vi "Receive Page.vi"(8 "error in (no error)":errorcluster, 11 "Node Ptr":T1 format="%.0x") -> (0 "error out":errorcluster)   [LabVIEW 2018, in "Vires VTD System Explorer.lvlib"]
uses:
  Vires VTD System Explorer.lvlib
  <vilib>/NI Veristand/Custom Device API/Custom Device Item Ref.ctl
  <vilib>/NI Veristand/Custom Device API/Custom Device Channel.ctl
  <vilib>/NI Veristand/Custom Device API/Custom Device Channel Type.ctl
  Shared/Constants.vi
  <vilib>/NI Veristand/Custom Device API/Custom Device API.lvlib
  Shared/Vires VTD Shared.lvlib
panel:
  in  "PlayerID":u8=1
  in  "RDB Receive Objects":string caption="RDB Object Name"
  in  "Add to Outputs":bool
  in  "Tree":string(tree)
  in  "Header":cluster{"Section Name":string}={"Section Name"="Custom Device Item Settings"}
  in  "Description":string
  in  "Name":string
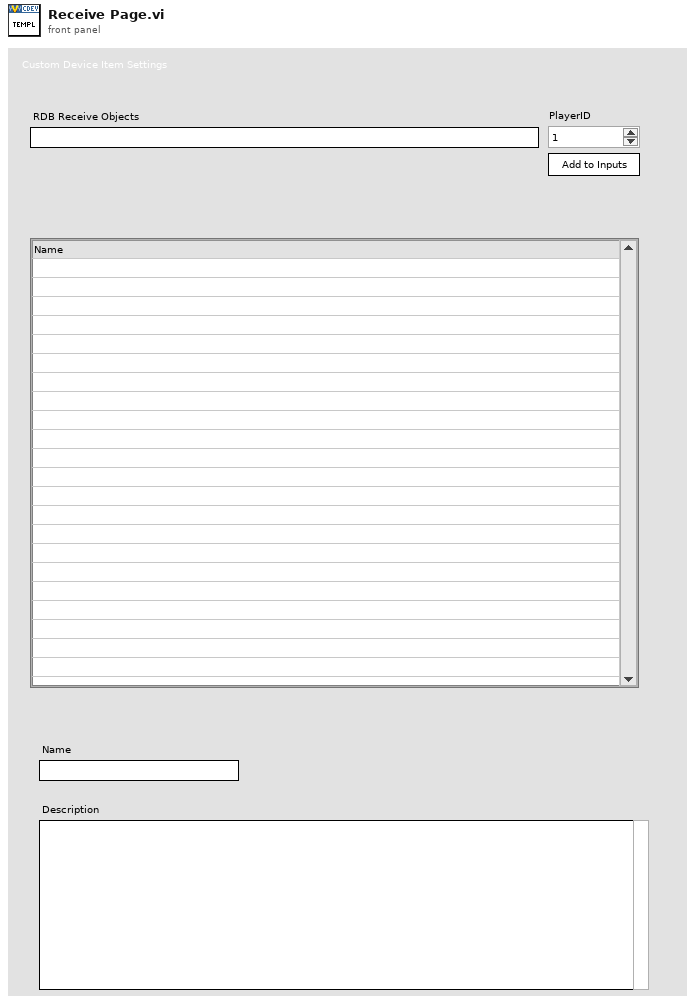
[diagram p1: front panel]
types:
  T1 = typedef "Custom Device API.lvlib/Custom Device Item Ref.ctl" = u64
  T2 = typedef "Custom Device API.lvlib/Custom Device Item Info.ctl" = cluster{"Name":string, "Is Channel":bool, "GUID":string, "Is Waveform":bool}
  T3 = typedef "Custom Device API.lvlib/Custom Device Channel.ctl" = cluster{"Type":T4, "Units":string, "Default Value":dbl, "Faultable":bool, "Scalable":bool}
  T4 = typedef "Custom Device API.lvlib/Custom Device Channel Type.ctl" = enum16{"Input", "Output"}
  T5 = typedef "Custom Device API.lvlib/Custom Device Commands.ctl" = enum16{"Default", "Item renamed", "Shutdown", "Dynamic button pressed"}
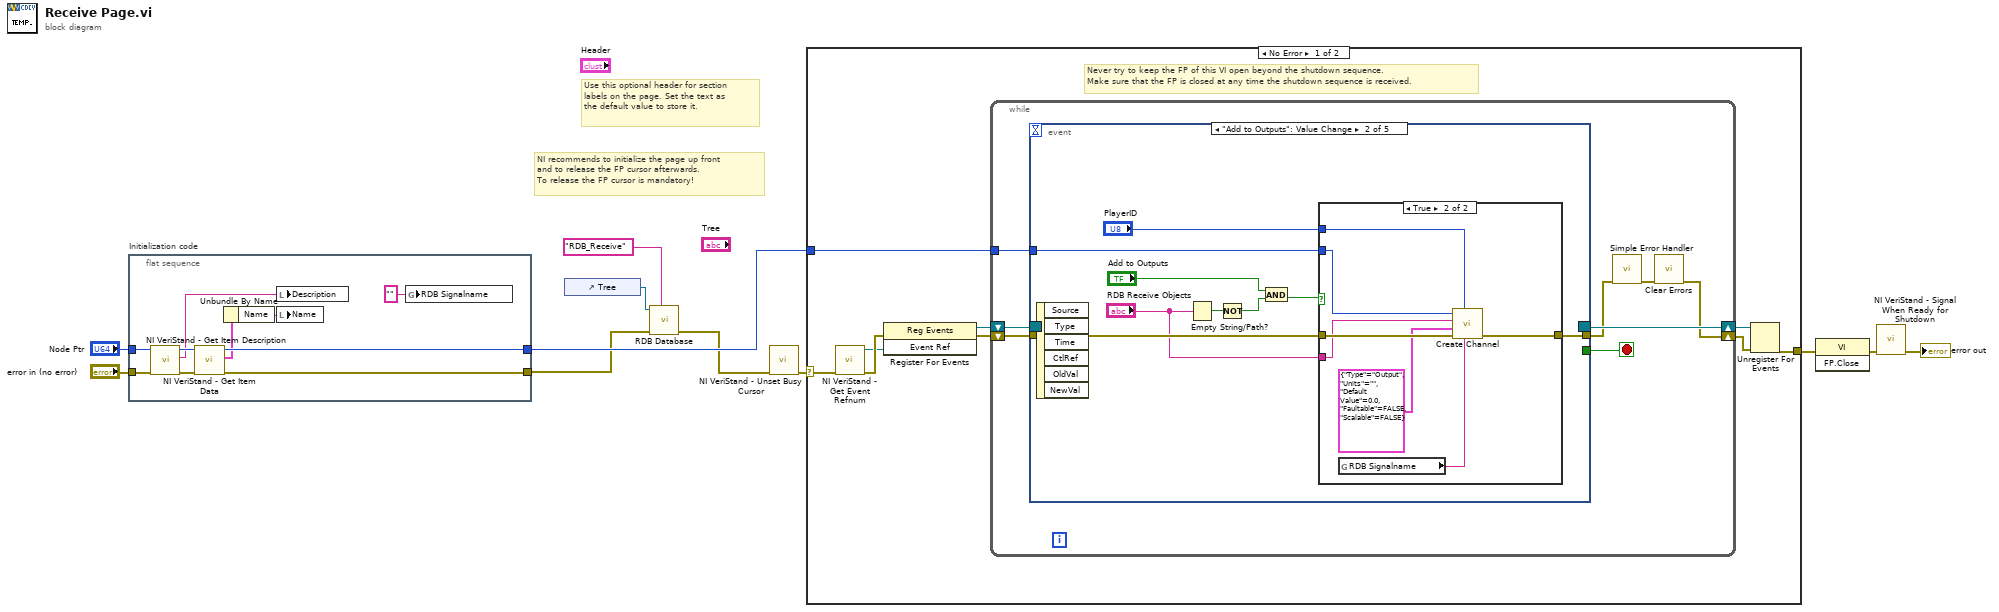
[diagram p0: block diagram]
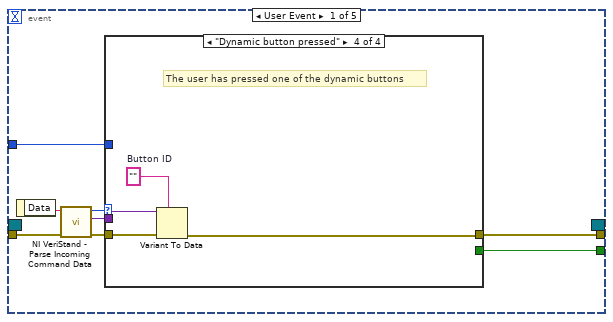
[diagram p2: hidden frame]
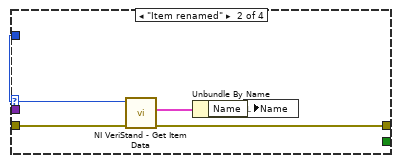
[diagram p4: hidden frame]
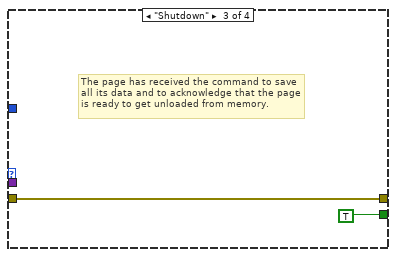
[diagram p5: hidden frame]
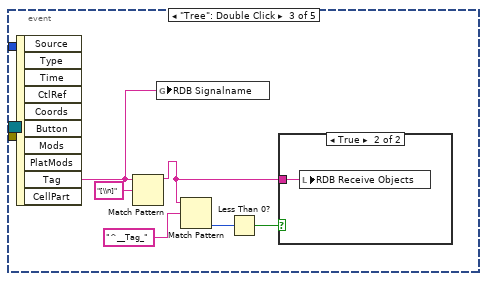
[diagram p7: hidden frame]
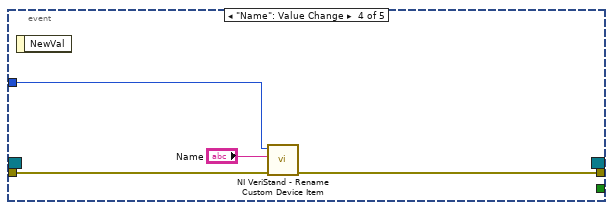
[diagram p9: hidden frame]
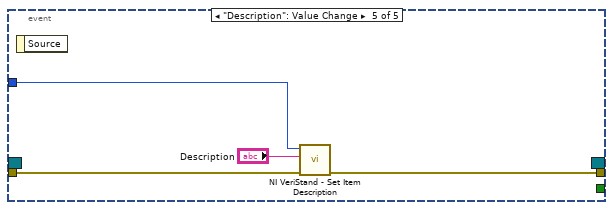
[diagram p10: hidden frame]
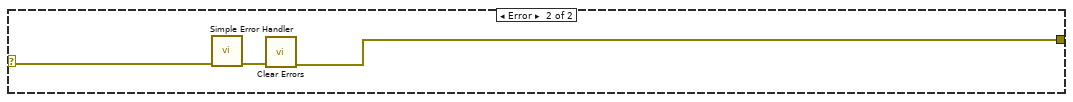
[diagram p11: hidden frame]
diagram:
  # "Use this optional header for section labels on the page. Set the text as the default value to store it."
  # "NI recommends to initialize the page up front\nand to release the FP cursor afterwards.\nTo release the FP cursor is mandatory!"
  n1 = flat-sequence "Initialization code" {
    tunnel: "error in (no error)" -> [w19]
    tunnel: "Node Ptr" -> [w18]
    tunnel: [w13] -> w4
    tunnel: [w21] -> w5
    frame #0 {
      n2 = call <vilib>:"NI VeriStand - Get Item Description.vi"("error in (no error)"=w19, "Item Ref in"=w18) -> ("error out"=w16:errorcluster, "Description"=w17:string, "Item Ref out"=w20:T1)  [unwired: 7 out]
      n3 = call <vilib>:"NI VeriStand - Get Item Data.vi"("error in (no error)"=w16, "Item Ref in"=w20) -> ("error out"=w13:errorcluster, "Item Info"=w15:T2, "Item Ref out"=w21:T1)  [unwired: 7 out]
      n4 = Unbundle By Name(w15) -> ("Name"=w14:string)
      n5 = local write "Description"(w17) -> ()
      n6 = local write "Name"(w14) -> ()
      n7 = global write "Constants.vi" "RDB Signalname"("" ("RDB Signalname")) -> ()
    }
  }
  n8 = control-ref of="Tree"() -> (w3:refnum<vi>)
  n9 = call "RDB Database.vi"("Filter Cluster"="RDB_Receive", "error in (no error)"=w4, "reference"=w3) -> ("error out"=w2:errorcluster)  [unwired: 8 in]
  n10 = call <vilib>:"NI VeriStand - Unset Busy Cursor.vi"("error in (no error)"=w2) -> ("error out"=w7:errorcluster)  [unwired: 10 out]
  n11 = case shown="No Error" w7 {
    selector: w7 -> [w22 w93]
    tunnel: [w27 w91] -> w11
    tunnel: w5 -> [w23 _]
    frame No Error {
      # "Never try to keep the FP of this VI open beyond the shutdown sequence.\nMake sure that the FP is closed at any time the shutdown sequence is received."
      n12 = call <vilib>:"NI VeriStand - Get Event Refnum.vi"("error in (no error)"=w22) -> ("error out"=w30:errorcluster, "Event Ref"=w26:refnum<user-event>)  [unwired: 9 out]
      n13 = register-events(error in=w30, w26) -> (reference out=w24:refnum<event-registration>, error out=w25:errorcluster)  [unwired: 1 in]
      n14 = while {
        tunnel: w23 -> [w34]
        shift-right: [w31] -> w28
        shift-left: w25 -> [w37]
        shift-right: [w38] -> w29
        shift-left: w24 -> [w36]
        stop <- w35 stop-if-true
        n15 = event shown="[1] \"Add to Outputs\": Value Change" {
          selector: w36 -> [_ _ _ _ _]
          dyn-events: [_ _ _ _ _] -> w38
          timeout: _ -> [_ _ _ _ _]
          tunnel: w37 -> [w46 w62 _ w86 w89]
          tunnel: [w42 _ _ _ _] -> w35
          tunnel: [w41 w60 _ w85 w88] -> w33
          tunnel: w34 -> [w40 w63 _ w84 w90]
          event User Event {
            n16 = event-data() -> ("Data"=w45:string)  [unwired: 1 out]
            n17 = call <vilib>:"NI VeriStand - Parse Incoming Command Data.vi"("error in (no error)"=w46, "Incoming data"=w45) -> ("error out"=w44:errorcluster, "Outgoing data"=w39:variant, "Action"=w43:T5)  [unwired: 7 out]
            n18 = case shown="\"Dynamic button pressed\"" w43 {
              tunnel: w44 -> [w47 w52 w53 w58]
              tunnel: [_ _ TRUE _] -> w42
              tunnel: [w47 w49 w53 w55] -> w41
              tunnel: w40 -> [_ w51 _ _]
              tunnel: w39 -> [_ _ _ w57]
              frame "Default", Default {
              }
              frame "Item renamed" {
                n19 = call <vilib>:"NI VeriStand - Get Item Data.vi"("error in (no error)"=w52, "Item Ref in"=w51) -> ("error out"=w49:errorcluster, "Item Info"=w50:T2)  [unwired: 8 out]
                n20 = Unbundle By Name(w50) -> ("Name"=w48:string)
                n21 = local write "Name"(w48) -> ()
              }
              frame "Shutdown" {
                # "The page has received the command to save all its data and to acknowledge that the page is ready to get unloaded from memory."
              }
              frame "Dynamic button pressed" {
                w56 = ""  # Button ID
                # "The user has pressed one of the dynamic buttons"
                n22 = Variant To Data(error in=w58, type=w56, Variant=w57) -> (error out=w55:errorcluster)  [unwired: 1 out]
              }
            }
          }
          event "Add to Outputs": Value Change {
            n23 = event-data() -> ()  [unwired: 7 out]
            n24 = Empty String/Path?(string/path="RDB Receive Objects") -> (empty?=w65:bool)
            n25 = Not(x=w65) -> (.not. x?=w66:bool)
            n26 = And(x="Add to Outputs", y=w66) -> (x .and. y?=w64:bool)
            n27 = case shown="True" w64 {
              tunnel: w63 -> [_ w75]
              tunnel: w62 -> [w68 w74]
              tunnel: "RDB Receive Objects" -> [_ w72]
              tunnel: [w68 w71] -> w60
              tunnel: "PlayerID" -> [_ w70]
              frame False {
              }
              frame True {
                n28 = global read "Constants.vi" "RDB Signalname"() -> (w69:string)
                n29 = call "Create Channel.vi"("RDB Signalname"=w69, "PlayerID"=w70, "error in (no error)"=w74, "Channel"=T3 {"Type"=enum."Output", "Units"="", "Default Value"=0.0, "Faultable"=FALSE, "Scalable"=FALSE}, "RDB Receive Objects"=w72, "Item Ref in"=w75) -> ("error out"=w71:errorcluster)  [unwired: 5 in]
              }
            }
          }
          event "Tree": Double Click {
            n30 = event-data() -> ("Tag"=w76:string)  [unwired: 10 out]
            n31 = Match Pattern(string=w76, regular expression="[\\n]") -> (before substring=w77:string)  [unwired: 1 in, 3 out]
            n32 = global write "Constants.vi" "RDB Signalname"(w76) -> ()
            n33 = Match Pattern(string=w77, regular expression="^__Tag_") -> (offset past match=w79:i32)  [unwired: 1 in, 3 out]
            n34 = Less Than 0?(x=w79) -> (x < 0?=w80:bool)
            n35 = case shown="True" w80 {
              tunnel: w77 -> [_ w82]
              frame False {
              }
              frame True {
                n36 = local write "RDB Receive Objects"(w82) -> ()
              }
            }
          }
          event "Name": Value Change {
            n37 = event-data() -> ()  [unwired: 2 out]
            n38 = call <vilib>:"NI VeriStand - Rename Custom Device Item.vi"("error in (no error)"=w86, "New Name"="Name", "Item Ref in"=w84) -> ("error out"=w85:errorcluster)  [unwired: 1 in, 7 out]
          }
          event "Description": Value Change {
            n39 = event-data() -> ()  [unwired: 2 out]
            n40 = call <vilib>:"NI VeriStand - Set Item Description.vi"("error in (no error)"=w89, "Description"="Description", "Item Ref in"=w90) -> ("error out"=w88:errorcluster)  [unwired: 8 out]
          }
        }
        n41 = call <vilib>:"Simple Error Handler.vi"("error in (no error)"=w33) -> ("error out"=w32:errorcluster)  [unwired: 1 in, 7 out]
        n42 = call <vilib>:"Clear Errors.vi"("error in (no error)"=w32) -> ("error out"=w31:errorcluster)  [unwired: 1 in, 5 out]
      }
      n43 = Unregister For Events(event registration refnum=w29, error in=w28) -> (error out=w27:errorcluster)
    }
    frame Error {
      n44 = call <vilib>:"Simple Error Handler.vi"("error in (no error)"=w93) -> ("error out"=w92:errorcluster)  [unwired: 1 in, 7 out]
      n45 = call <vilib>:"Clear Errors.vi"("error in (no error)"=w92) -> ("error out"=w91:errorcluster)  [unwired: 1 in, 5 out]
    }
  }
  n46 = invoke class="VI" method="FP.Close"(error in=w11) -> (error out=w10:errorcluster)  [unwired: 2 in, 2 out]
  n47 = call <vilib>:"NI VeriStand - Signal When Ready for Shutdown.vi"("error in (no error)"=w10) -> ("error out"=→"error out":errorcluster)  [unwired: 10 out]
